vi "Flag_Parse.vi"(8 "error in (no error)":errorcluster) -> (0 "error out":errorcluster, 2 "Stop?":bool, 3 "Pause?":bool)   [LabVIEW 2016, in "SeqProcessor.lvlib"]
uses:
  SeqProcessor.lvlib
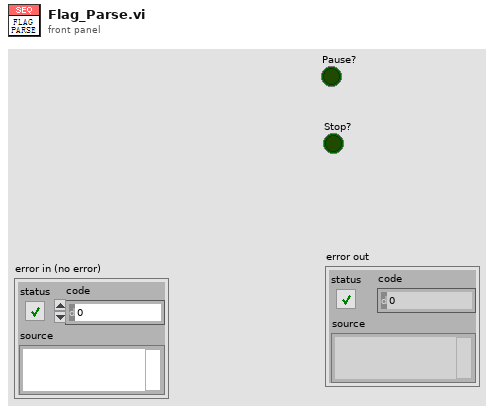
[diagram p1: front panel]
types:
  T1 = typedef "SeqProcessor.lvlib/Flag.ctl" = cluster{"SingleStep":bool, "Pause":bool, "Stop":bool, "StepbyStep":bool}
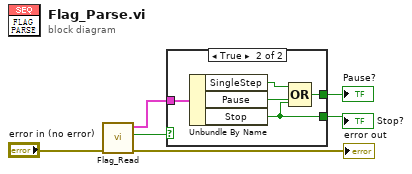
[diagram p0: block diagram]
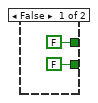
[diagram p2: hidden frame]
diagram:
  n1 = call "Flag_Read.vi"("error in (no error)"="error in (no error)") -> ("error out"=→"error out":errorcluster, "Found?"=w2:bool, "Flag"=w5:T1)  [unwired: 8 in]
  n2 = case shown="True" w2 {
    tunnel: w5 -> [_ w13]
    tunnel: [FALSE w10] -> w4
    tunnel: [FALSE ("Stop") w9] -> w3
    frame False {
    }
    frame True {
      n3 = Unbundle By Name(w13) -> ("SingleStep"=w12:bool, "Pause"=w11:bool, "Stop"=w9:bool)
      n4 = Compound Arithmetic op=OR(w12, w11, w9) -> (w10:bool)
    }
  }
  "Pause?" <- w4
  "Stop?" <- w3
